vi "Commit NVMEM Areas.vi"(0 "session in":refnum<k21>, 5 "NVMEM areas":refnum<k21>="$DefaultNVMEMAreas", 11 "error in (no error)":errorcluster) -> (4 "session out":refnum<k21>, 15 "error out":errorcluster)   [LabVIEW 2020, in "SLSC.lvlib"]
doc: "Commits pending changes to hardware for the specified NVMEM area(s). If you set the same address multiple times between commits, only the last value will be committed."
uses:
  <vilib>/SLSC/SLSC.lvlib
  nislsclvapi.dll
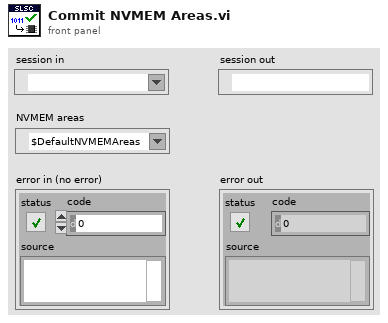
[diagram p1: front panel]
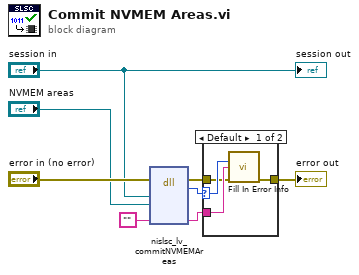
[diagram p0: block diagram]
diagram:
  n1 = dll-call lib="nislsclvapi.*" fn="nislsc_lv_commitNVMEMAreas"(error in="error in (no error)", "session"="session in", "nvmemAreas"="NVMEM areas", "extendedErrorInfo"="") -> (error out=w3:errorcluster, "return type"=w4:i32, "extendedErrorInfo"=w5:string)  [unwired: 6 in, 1 out]
  n2 = case shown="Default" w4 {
    selector: w4 -> [w12 _]
    tunnel: w5 -> [w11 _]
    tunnel: w3 -> [w10 w13]
    tunnel: [w9 w13] -> w2
    frame Default {
      n3 = call <vilib>:"Fill In Error Info.vi"("status code"=w12, "extended error info"=w11, "error in"=w10) -> ("error out"=w9:errorcluster)  [unwired: 12 in]
    }
    frame 0 {
    }
  }
  "error out" <- w2
  "session out" <- "session in"
